vi "get_config_cluster.vi"(8 "error in (no error)":errorcluster, 11 "GenericPlugin in":refnum<class "SweepDL090926Automation.lvclass">) -> (0 "error out":errorcluster, 2 "config cluster (variant)":variant, 3 "GenericPlugin out":refnum<class "SweepDL090926Automation.lvclass">)   [LabVIEW 2010, in "SweepDL090926Automation.lvclass"]
uses:
  SweepDL090926Automation.lvclass
  SweepDL090926Automation.lvclass/SweepDL090926Automation.ctl
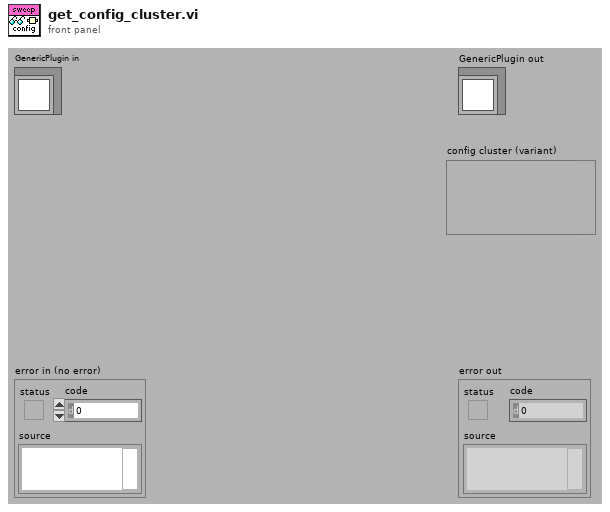
[diagram p1: front panel]
types:
  T1 = typedef "SweepDL090926Automation.lvclass/config_data_cluster.ctl" = cluster{"imaging-mode sequence":T2[]}
  T2 = typedef "plugin_specification.ctl" = cluster{"class path":string, "configuration":string, "label":string, "settings name":string}
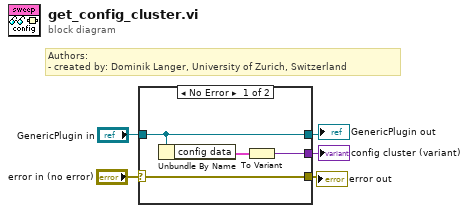
[diagram p0: block diagram]
diagram:
  # "Authors: \n- created by: Dominik Langer, University of Zurich, Switzerland"
  n1 = case shown="No Error" "error in (no error)" {
    selector: "error in (no error)" -> [w9 w10]
    tunnel: "GenericPlugin in" -> [w8 w11]
    tunnel: [w9 w10] -> w2
    tunnel: [w8 w11] -> w1
    tunnel: [w6 _] -> w3
    frame No Error {
      n2 = Unbundle By Name(w8) -> ("config data"=w7:T1)
      n3 = To Variant(anything=w7) -> (Variant=w6:variant)
    }
    frame Error {
    }
  }
  "error out" <- w2
  "GenericPlugin out" <- w1
  "config cluster (variant)" <- w3
